vi "Wiimote Parse Core Buttons.vi"(8 "error in":errorcluster, 11 "pReportBuffer in":u8[](array[numeric]) format="%02x") -> (0 "error out":errorcluster, 3 "Wiimote Buttons out":T1)   [LabVIEW 2012, in "Wiimote.lvlib"]
uses:
  Wiimote.lvlib
  Wiimote Buttons.ctl
panel:
  in  "Wiimote Buttons in":T1
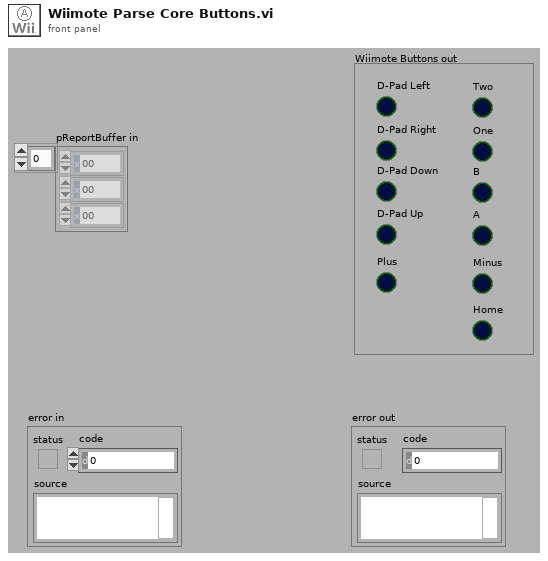
[diagram p1: front panel]
types:
  T1 = typedef "Wiimote.lvlib/Wiimote Buttons.ctl" = cluster{"D-Pad Left":bool, "D-Pad Right":bool, "D-Pad Down":bool, "D-Pad Up":bool, "Plus":bool, "Two":bool, "One":bool, "B":bool, "A":bool, "Minus":bool, "Home":bool}
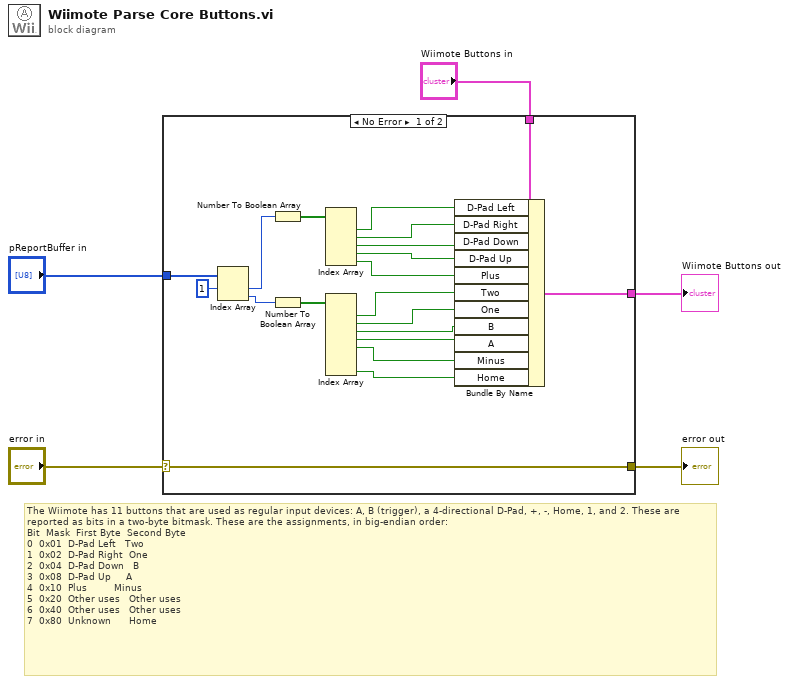
[diagram p0: block diagram]
diagram:
  # "The Wiimote has 11 buttons that are used as regular input devices: A, B (trigger), a 4-directional D-Pad, +, -, Home, 1, and 2. These are reported as bits in a two-byte bitmask. These are the assignments, in big-endian order:\nBit \tMask \tFirst Byte \tSecond Byte\n0 \t0x01 \tD-Pad Left \t Two\n1 \t0x02 \tD-Pad Right \tOne\n2 \t0x04 \tD-Pad Down \t B\n3 \t0x08 \tD-Pad Up \t   A\n4 \t0x10 \tPlus \t       Minus\n5 \t0x20 \tOther uses \t Other uses\n6 \t0x40 \tOther uses \t Other uses\n7 \t0x80 \tUnknown \t    Home"
  n1 = case shown="No Error" "error in" {
    selector: "error in" -> [w25 w26]
    tunnel: [w25 w26] -> w4
    tunnel: "pReportBuffer in" -> [w22 _]
    tunnel: "Wiimote Buttons in" -> [w19 _]
    tunnel: [w7 _] -> w1
    frame No Error {
      n2 = Index Array(array=w22, index #1=1 ("index")) -> (element #1=w24:u8, element #2=w21:u8)  [unwired: 1 in]
      n3 = Number To Boolean Array(number=w24) -> (Boolean array=w20:bool[])
      n4 = Number To Boolean Array(number=w21) -> (Boolean array=w13:bool[])
      n5 = Index Array(array=w20) -> (element #1=w18:bool, element #2=w17:bool, element #3=w16:bool, element #4=w15:bool, element #5=w14:bool)  [unwired: 5 in]
      n6 = Index Array(array=w13) -> (element #1=w12:bool, element #2=w11:bool, element #3=w10:bool, element #4=w9:bool, element #5=w8:bool, element #8=w6:bool)  [unwired: 8 in, 2 out]
      n7 = Bundle By Name(cluster=w19, "D-Pad Left"=w18, "D-Pad Right"=w17, "D-Pad Down"=w16, "D-Pad Up"=w15, "Plus"=w14, "Two"=w12, "One"=w11, "B"=w10, "A"=w9, "Minus"=w8, "Home"=w6) -> (w7:T1)
    }
    frame Error {
    }
  }
  "error out" <- w4
  "Wiimote Buttons out" <- w1
